vi "Remove.vi"(8 "error in (no error)":errorcluster caption="错误输入（无错误）", 10 "Key":string, 11 "Dictionary In":refnum<class "Dictionary.lvclass"> caption="DNL_LabVIEW Object in") -> (0 "error out":errorcluster caption="错误输出", 1 "Key Exist?":bool, 2 "Removed Value":string, 3 "Dictionary Out":refnum<class "Dictionary.lvclass"> caption="DNL_LabVIEW Object out")   [LabVIEW 2012, in "Dictionary.lvclass"]
uses:
  Dictionary.lvclass
  Dictionary.lvclass/Dictionary.ctl
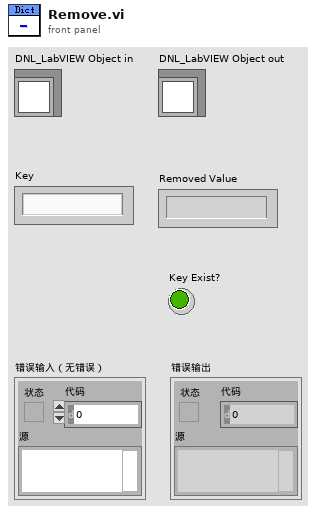
[diagram p1: front panel]
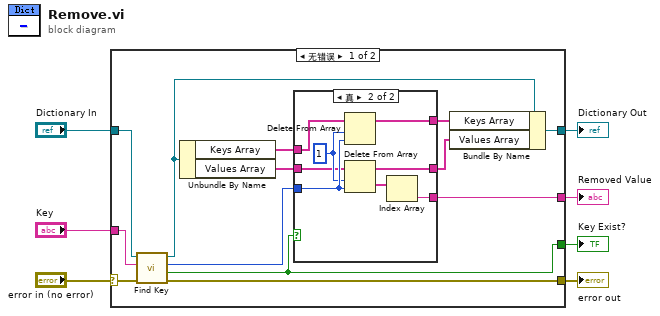
[diagram p0: block diagram]
diagram:
  n1 = case shown="无错误" "error in (no error)" {
    selector: "error in (no error)" -> [w19 w32]
    tunnel: [w18 w32] -> w6
    tunnel: [w9 w31] -> w4
    tunnel: "Dictionary In" -> [w20 w31]
    tunnel: "Key" -> [w17 _]
    tunnel: [w13 _] -> w1
    tunnel: [w8 _] -> w2
    frame No Error {
      n2 = call "Find Key.vi"("error in (no error)"=w19, "Key"=w17, "Dictionary In"=w20) -> ("error out"=w18:errorcluster, "Key Exist?"=w8:bool, "Index"=w16:i32, "Dictionary Out"=w12:refnum<class "Dictionary.lvclass">)  [unwired: 5 in]
      n3 = Unbundle By Name(w12) -> ("Keys Array"=w15:string[], "Values Array"=w14:string[])
      n4 = case shown="真" w8 {
        tunnel: w16 -> [_ w30]
        tunnel: w15 -> [w22 w28]
        tunnel: w14 -> [w21 w27]
        tunnel: [w22 w26] -> w11
        tunnel: [w21 w25] -> w10
        tunnel: [_ w23] -> w13
        frame False {
        }
        frame True {
          w29 = 1 ("长度")
          n5 = Delete From Array(array=w28, length=w29, index=w30) -> (array with subset deleted=w26:string[])  [unwired: 1 out]
          n6 = Delete From Array(array=w27, length=w29, index=w30) -> (deleted portion=w24:string[], array with subset deleted=w25:string[])
          n7 = Index Array(array=w24) -> (element=w23:string)  [unwired: 1 in]
        }
      }
      n8 = Bundle By Name(cluster=w12, "Keys Array"=w11, "Values Array"=w10) -> (w9:refnum<class "Dictionary.lvclass">)
    }
    frame Error {
    }
  }
  "error out" <- w6
  "Dictionary Out" <- w4
  "Key Exist?" <- w2
  "Removed Value" <- w1
